vi "OCT Motor Ctrl.vi"() -> ()   [LabVIEW 2016]
uses:
  <vilib>/Platform/TimedLoop/XDataNode/timing_clust.ctl
  <vilib>/Platform/TimedLoop/XDataNode/nitl_modes.ctl
  <vilib>/Platform/TimedLoop/XDataNode/wakeup.ctl
  <vilib>/FPGAPlugInAG/PXI-7833R/niLvFpga_Open_PXI-7833R.vi
  <vilib>/Utility/error.llb/Error Cluster From Error Code.vi
  <vilib>/rvi/errors/niLvFpgaAdjustHostInterfaceError.vi
  <vilib>/platform/TimedLoop/XDataNode/XDataNode.xnode
  <vilib>/rvi/interface/nirviOpenFPGA/nirviOpenFPGA.xnode
  FPGA Bitfiles/PhantomControlPI_FPGATarget_QuadCtr2_E2412E44.lvbitx
  IRISS_FPGA_IO.vi
  <vilib>/rvi/interface/nirviReadWriteControl/nirviReadWriteControl.xnode
  <vilib>/Platform/TimedLoop/XDataNode/XDNodeRunTimeDep.lvlib
  Library/jmslib.lvlib
  NiFpgaLv.dll
panel:
  in  "Threshold (cnts)":dbl=500.0
  out "Knob Enc Position (mm)":dbl
  out "Waveform Chart":cluster{"Reference":dbl, "Position OCT Mot":i32}(graph)
  in  "Reference (mm)":dbl step=0.5
  in  "Motor On":bool=TRUE
  in  "PID Gains":cluster{"Kp":dbl, "Kd":dbl, "Ki":dbl}={"Kp"=0.0003, "Kd"=0.0, "Ki"=0.01} {"Kp" min=0.0 step=0.0001}
  in  "stop":bool
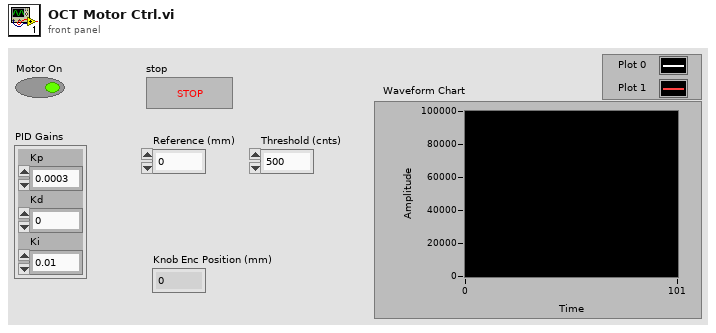
[diagram p1: front panel]
types:
  T1 = typedef "XDNodeRunTimeDep.lvlib/timing_clust.ctl" = cluster{"Expected End [f-1]":u64, "Actual End [f-1]":u64, "Finished Late? [f-1]":bool, "Expected End [i-1]":u64, "Actual End [i-1]":u64, "Finished Late? [i-1]":bool, "Expected Start [i]":u64, "Actual Start [i]":u64, "Expected Start [f]":u64, "Actual Start [f]":u64, "Source Name":string, "Structure Name":string, "Period":i64, "Deadline":i64, "Offset":i64, "Start":i64, "Priority":i32, "Timeout":i32, "Mode":T2, "Wakeup Reason":T3, "Error":errorcluster, "Source Type":string, "Secondary Source Type":string, "Global End Time":u64, "Global Start Time":u64, "Frame Duration":u64, "Iteration Duration":u64, "Assigned CPU":i32, "I/O Scan Engine Mode":u32}
  T2 = typedef "XDNodeRunTimeDep.lvlib/nitl_modes.ctl" = enum32{"No Change", "Process missed periods, maintain original phase", "Discard missed periods, maintain original phase", "Process missed periods, ignore original phase", "Discard missed periods, ignore original phase"}
  T3 = typedef "XDNodeRunTimeDep.lvlib/wakeup.ctl" = enum32{"Normal", "Aborted", "Asynchronous wakeup", "Timing source error", "Timed loop error", "Timeout"}
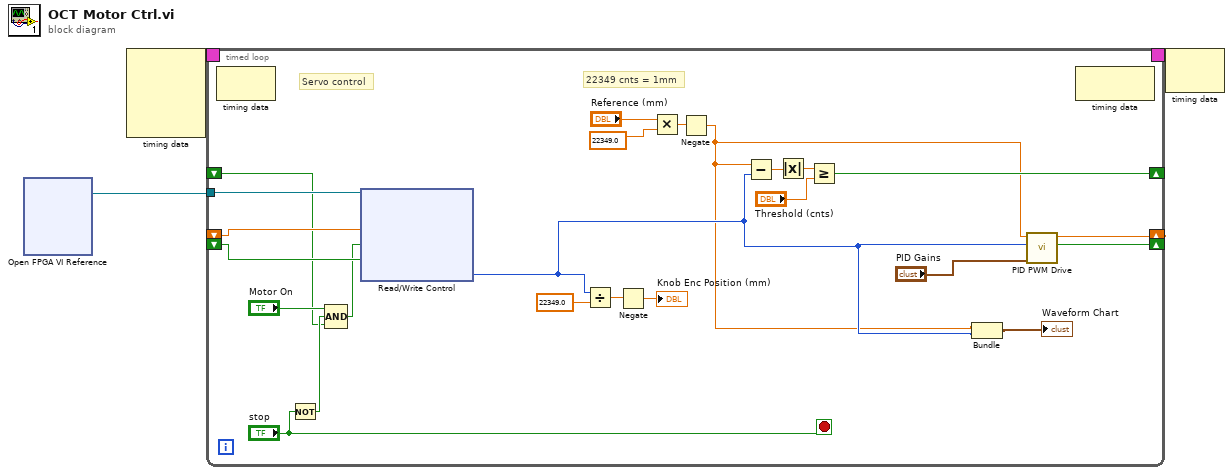
[diagram p0: block diagram]
diagram:
  n1 = xnode "Open FPGA VI Reference"() -> ("FPGA VI Reference Out"=w1:refnum<k20>)  [unwired: 2 in, 1 out]
  n2 = node-c288() -> (w3:T1)  [unwired: 4 in]
  n3 = timed-loop {
    timing: w3 -> [_]
    timing-out: [_] -> w2
    tunnel: w1 -> [w27]
    shift-right: [w25] -> _
    shift-left: _ -> [w23]
    shift-right: [w24] -> _
    shift-left: _ -> [w22]
    shift-right: [w15] -> _
    shift-left: _ -> [w14]
    stop <- "stop" stop-if-true
    # "22349 cnts = 1mm"
    # "Servo control"
    n4 = node-c288() -> ()  [unwired: 1 in, 1 out]
    n5 = Not(x="stop") -> (.not. x?=w19:bool)
    n6 = Compound Arithmetic op=AND("Motor On", w19, w14) -> (w13:bool)
    n7 = xnode "Read/Write Control"("FPGA VI Reference In"=w27, "OCT Mot DC"=w23, "INHB OCT Mot"=w13, "DIR OCT Mot"=w22) -> ("32 bit Position 14"=w8:i32)  [unwired: 1 in, 3 out]
    n8 = Divide(x=w8, y=22349.0) -> (x/y=w5:dbl)
    n9 = Negate(x=w5) -> (-x=→"Knob Enc Position (mm)":dbl)
    n10 = Multiply(x="Reference (mm)", y=22349.0) -> (x*y=w7:dbl)
    n11 = Negate(x=w7) -> (-x=w6:dbl)
    n12 = Subtract(x=w6, y=w8) -> (x-y=w17:dbl)
    n13 = Absolute Value(x=w17) -> (abs(x)=w16:dbl)
    n14 = Greater Or Equal?(x=w16, y="Threshold (cnts)") -> (x >= y?=w15:bool)
    n15 = Bundle(w6, "32 bit Position 14"=w8) -> (→"Waveform Chart":cluster{dbl, "32 bit Position 14":i32})  [unwired: 1 in]
    n16 = call "PID PWM Drive.vi"("PID Gains"="PID Gains", "Encoder Position"=w8, "Reference"=w6) -> ("Direction"=w24:bool, "Duty Cycle"=w25:dbl)  [unwired: 6 in, 1 out]
    n17 = node-c288() -> ()  [unwired: 1 in, 1 out]
  }
  n18 = node-c288(w2) -> ()  [unwired: 1 out]
